vi "d calc w y finish.vi"(4 "YP":dbl) -> (0 "d":dbl)   [LabVIEW 2016]
uses:
  Program Files (x86)/National Instruments/LabVIEW 2016/examples/FRC/roboRIO/Vision/2017 Vision Example/Vision Support Code/Camera Types.ctl
panel:
  in  "Camera Type":T1
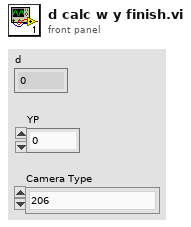
[diagram p1: front panel]
types:
  T1 = typedef "Camera Types.ctl" = enum16{"206", "1011", "1013", "MS HD3000 square", "MS HD3000 640x480"}
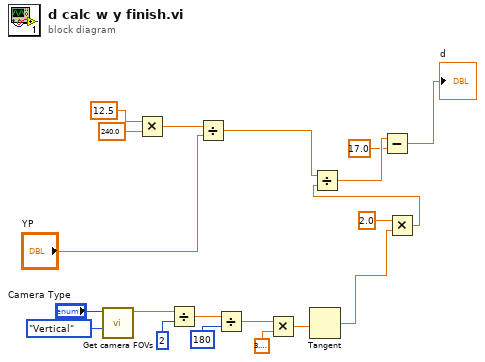
[diagram p0: block diagram]
diagram:
  n1 = call "Get camera FOVs.vi"("Type"=enum16{"Horizontal", "Vertical", "Diagonal"}."Vertical" ("Angle"), "Camera Type"="Camera Type") -> ("FOV"=w9:dbl)  [unwired: 8 in, 1 out]
  n2 = Multiply(x=12.5, y=240.0) -> (x*y=w18:dbl)
  n3 = Divide(x=w9, y=2) -> (x/y=w12:dbl)
  n4 = Divide(x=w18, y="YP") -> (x/y=w16:dbl)
  n5 = Divide(x=w12, y=180) -> (x/y=w11:dbl)
  n6 = Multiply(x=w11, y=3.141592653589793) -> (x*y=w13:dbl)
  n7 = Tangent(1:w13) -> (0:w6:dbl)
  n8 = Multiply(x=2.0, y=w6) -> (x*y=w4:dbl)
  n9 = Divide(x=w16, y=w4) -> (x/y=w3:dbl)
  n10 = Subtract(x=w3, y=17.0) -> (x-y=→"d":dbl)
